vi "Read_pH.vi"(11 "pH sensor Channel":tag) -> (0 "pH value":dbl, 1 "after":dbl(knob) scale=0.0..5.0, 2 "ph":dbl(knob) scale=0.0..14.0, 3 "before":dbl(knob) scale=0.0..5.0)   [LabVIEW 2022 SP3]
uses:
  <vilib>/DAQmx/miscellaneous.llb/DAQmx Fill In Error Info.vi
  <vilib>/DAQmx/create/channels.llb/DAQmx Create Channel (AI-Voltage-Basic).vi
  <vilib>/ptbypt/NI_PtbyPt.lvlib
  <vilib>/DAQmx/read.llb/DAQmx Read (Analog DBL 1Chan 1Samp).vi
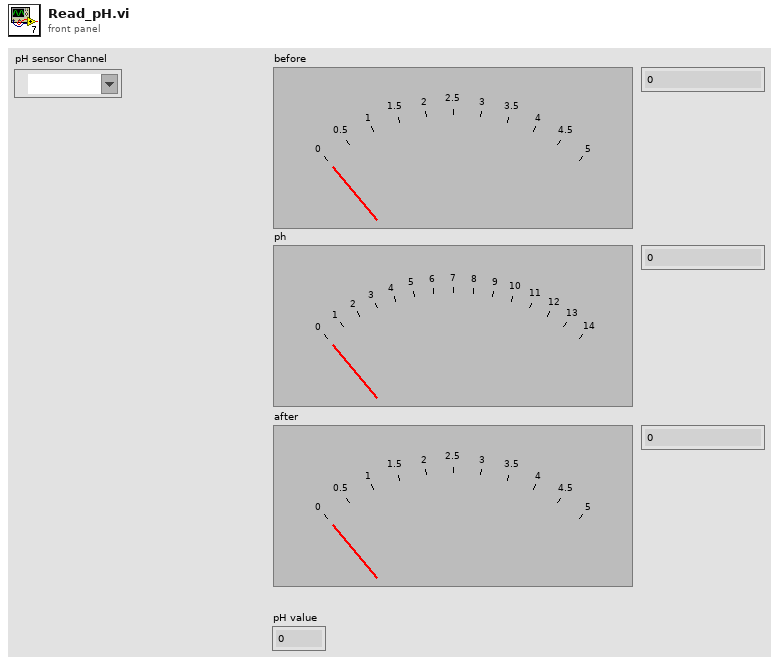
[diagram p1: front panel]
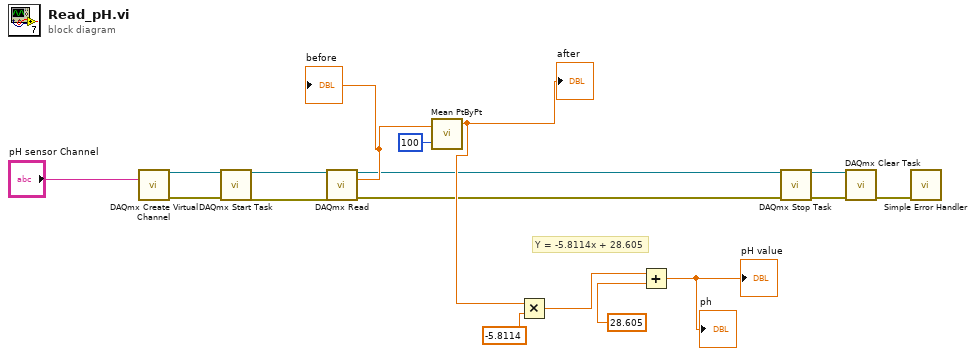
[diagram p0: block diagram]
diagram:
  # "Y = -5.8114x + 28.605"
  n1 = call-poly <vilib>:"DAQmx Create Virtual Channel.vi"("physical channels"="pH sensor Channel") -> ("task out"=w13:refnum<k21>, "error out"=w12:errorcluster)  [unwired: 13 in]
  n2 = call <vilib>:"DAQmx Start Task.vi"("task/channels in"=w13, "error in"=w12) -> ("task out"=w5:refnum<k21>, "error out"=w4:errorcluster)  [unwired: 12 in]
  n3 = call-poly <vilib>:"DAQmx Read.vi"("task/channels in"=w5, "error in"=w4) -> ("task out"=w3:refnum<k21>, "data"=w8:dbl, "error out"=w2:errorcluster)  [unwired: 11 in]
  "before" <- w8
  n4 = call <vilib>:"Mean PtByPt.vi"("x"=w8, "sample length"=100) -> ("mean"=w7:dbl)  [unwired: 2 in, 1 out]
  "after" <- w7
  n5 = Multiply(x=w7, y=-5.8114) -> (x*y=w6:dbl)
  n6 = Add(x=w6, y=28.605) -> (x+y=→"ph" →"pH value":dbl)
  n7 = call <vilib>:"DAQmx Stop Task.vi"("task/channels in"=w3, "error in"=w2) -> ("task out"=w16:refnum<k21>, "error out"=w15:errorcluster)  [unwired: 12 in]
  n8 = call <vilib>:"DAQmx Clear Task.vi"("task in"=w16, "error in"=w15) -> ("error out"=w17:errorcluster)  [unwired: 13 in]
  n9 = call <vilib>:"Simple Error Handler.vi"("error in (no error)"=w17) -> ()  [unwired: 4 in, 5 out]
